vi "14.2 Bottle Check.vi"(8 "ErrI":errorcluster) -> (0 "ErrO":errorcluster)   [LabVIEW 2016]
uses:
  <vilib>/vision/Measure.llb/Straight Edge Options.ctl
  <vilib>/vision/Measure.llb/Straight Edge Process.ctl
  <vilib>/vision/Image Controls.llb/IMAQ Image.ctl
  <vilib>/vision/Measure.llb/Edge Options.ctl
  <vilib>/vision/Measure.llb/Edge Polarity.ctl
  <vilib>/vision/NI_Vision_Development_Module.lvlib
panel:
  out "Pass?":bool
  out "Liquied Level":dbl format="%.2f"
  in  "Line Fit Options":T1={"Number of Lines"=1, "Type"=enum."Best Edge Rake", "Min. Score"=10.0, "Max. Score"=1000.0, "Orientation"=0.0, "Angle Range"=45.0, "Angle Tolerance"=1.0, "Step Size"=7, "Min. SNR (db)"=0.0, "Min. Points (%)"=25.0, "Hough Iterations"=5} {"Min. Points (%)" min=0.0 max=100.0; "Min. SNR (db)" min=0.0; "Max. Score" min=0.0 max=1024.0; "Min. Score" min=0.0 max=1024.0 step=1.0}
  out "Image":T3(plugin-control)
  in  "Next":bool
  in  "Exit":bool
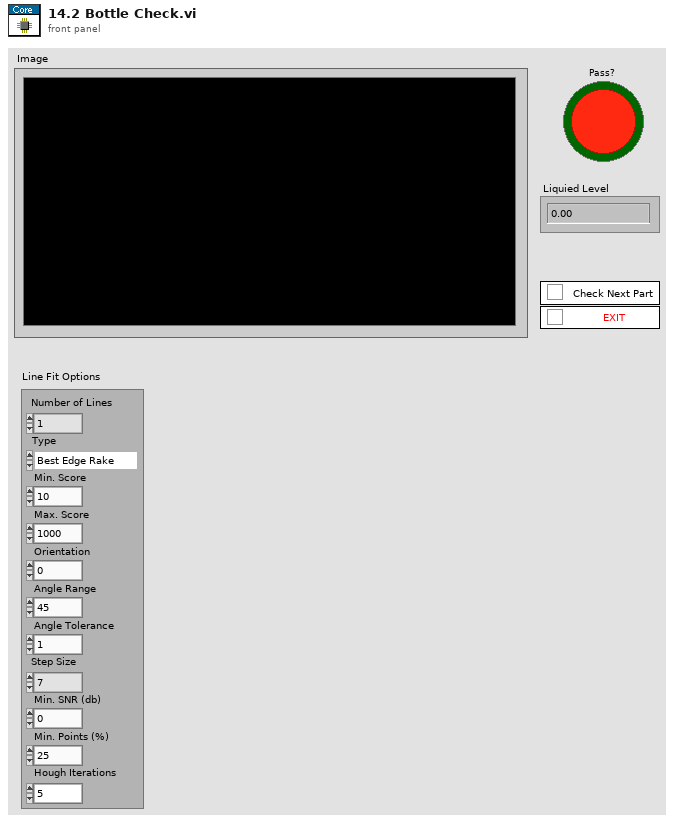
[diagram p1: front panel]
types:
  T1 = typedef "Straight Edge Options.ctl" = cluster{"Number of Lines":i32, "Type":T2, "Min. Score":dbl, "Max. Score":dbl, "Orientation":dbl, "Angle Range":dbl, "Angle Tolerance":dbl, "Step Size":u32, "Min. SNR (db)":dbl, "Min. Points (%)":dbl, "Hough Iterations":i32}
  T2 = typedef "Straight Edge Process.ctl" = enum32{"First Edge Rake", "Best Edge Rake", "Hough Edge Rake", "First Edge Projection", "Best Edge Projection"}
  T3 = typedef "IMAQ Image.ctl" = refnum<image>
  T4 = typedef "IMAQ Rectangle" = cluster{"Left":i32, "Top":i32, "Right":i32, "Bottom":i32, "Rotation":dbl}
  T5 = cluster{"Point1":cluster{"X":sgl, "Y":sgl}, "Point2":cluster{"X":sgl, "Y":sgl}}
  T6 = typedef "IMAQ Coordinate System" = cluster{"Reference System":cluster{"Origin":cluster{"X":sgl, "Y":sgl}, "Angle (deg)":sgl, "Axis Reference":u32}, "Measurement System":cluster{"Origin":cluster{"X":sgl, "Y":sgl}, "Angle (deg)":sgl, "Axis Reference":u32}}
  T7 = cluster{"Src":T3, "Dst":T3, "Parts":string[], "RefCoord":T6, "MsrCoord":T6, "MsrROI":T4, "RefLine":cluster{"Point1":cluster{"X":sgl, "Y":sgl}, "Point2":cluster{"X":sgl, "Y":sgl}}}
  T8 = typedef "Edge Options.ctl" = cluster{"Edge Polarity":T9, "Kernel Size":u32, "Width":u32, "Minimum Edge Strength":sgl, "Interpolation Type":enum32{"Zero Order", "Bilinear", "Quadratic", "Cubic", "Bilinear Fixed"}, "Data Processing Method":enum32{"Average", "Median"}}
  T9 = typedef "Edge Polarity.ctl" = u32
  T10 = cluster{"Direction":u16, "Primary Edge Options":T8, "Secondary Edge Options":T8, "Show Search Area":bool, "Show Search Lines":bool, "Show Edges Found":bool, "Show Result":bool, "Search Area Color":u32, "Search Lines Color":u32, "Edge Locations Color":u32, "Result Color":u32, "Overlay Group Name":string}
  T11 = typedef "ROI Descriptor" = cluster{"Global Rectangle":i32[], "Contours":cluster{"ID":enum32{"External", "Internal"}, "Type":u32, "Coordinates":i32[]}[]}
  T12 = cluster{"Search Direction":u32, "Edge Options":T8, "Show Search Area":bool, "Show Search Lines":bool, "Show Edges Found":bool, "Show Result":bool, "Search Area Color":u32, "Search Lines Color":u32, "Edge Locations Color":u32, "Result Color":u32, "Overlay Group Name":string}
  T13 = cluster{"Point1 (Pixels)":cluster{"X":sgl, "Y":sgl}, "Point2 (Pixels)":cluster{"X":sgl, "Y":sgl}, "Point1 (Real-World)":cluster{"X":sgl, "Y":sgl}, "Point2 (Real-World)":cluster{"X":sgl, "Y":sgl}, "Angle (Pixel)":dbl, "Angle (Real-World)":dbl, "Score":dbl, "Straightness":dbl, "Average SNR (db)":dbl, "Calibration Valid":bool}[]
  T14 = cluster{"Point1 (Pixels)":cluster{"X":sgl, "Y":sgl}, "Point2 (Pixels)":cluster{"X":sgl, "Y":sgl}, "Point1 (Real-World)":cluster{"X":sgl, "Y":sgl}, "Point2 (Real-World)":cluster{"X":sgl, "Y":sgl}, "Angle (Pixel)":dbl, "Angle (Real-World)":dbl, "Score":dbl, "Straightness":dbl, "Average SNR (db)":dbl, "Calibration Valid":bool}
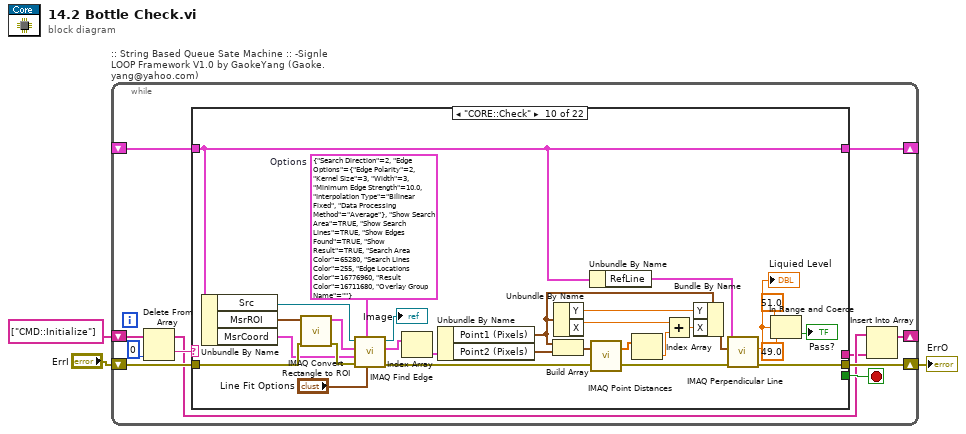
[diagram p0: block diagram]
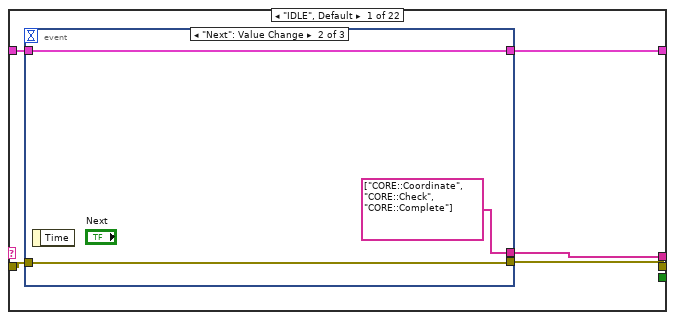
[diagram p2: hidden frame]
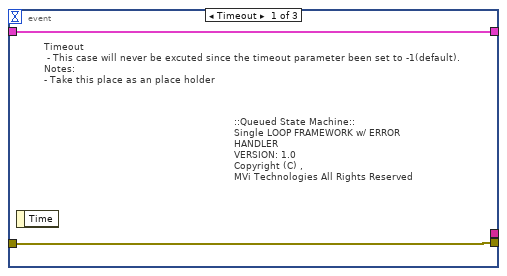
[diagram p3: hidden frame]
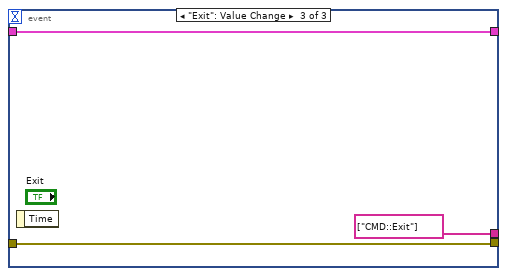
[diagram p4: hidden frame]
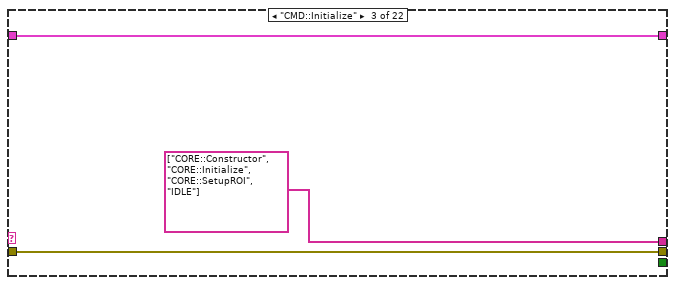
[diagram p6: hidden frame]
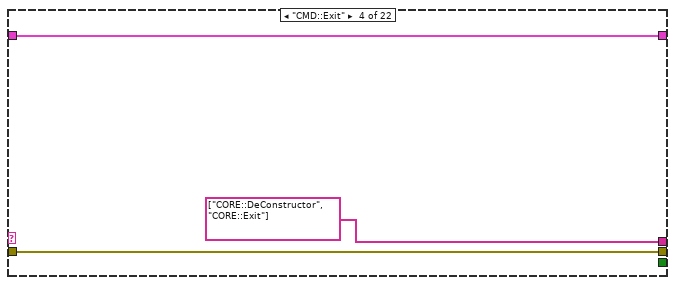
[diagram p7: hidden frame]
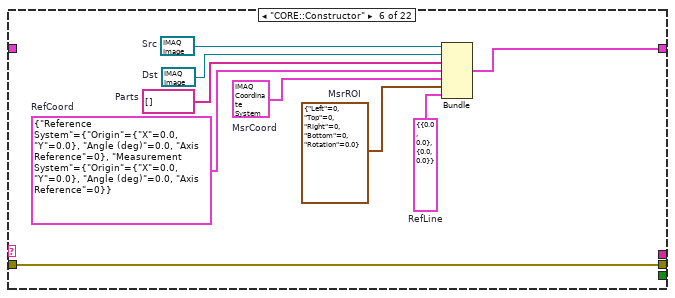
[diagram p9: hidden frame]
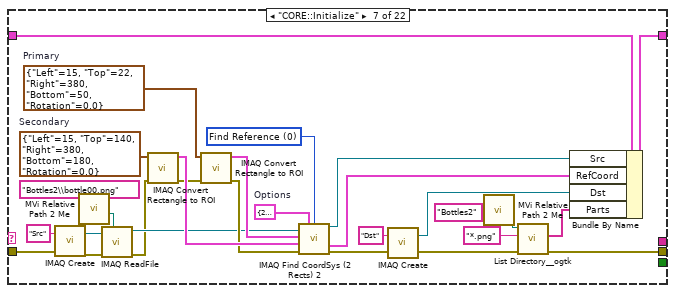
[diagram p10: hidden frame]
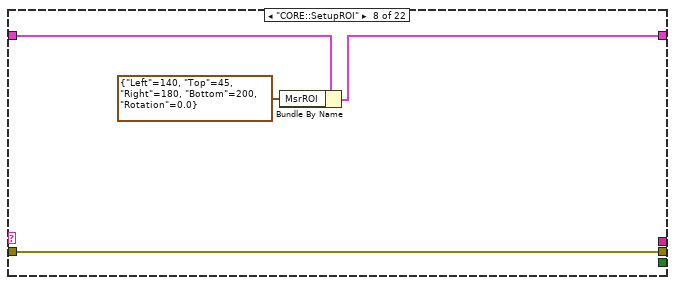
[diagram p11: hidden frame]
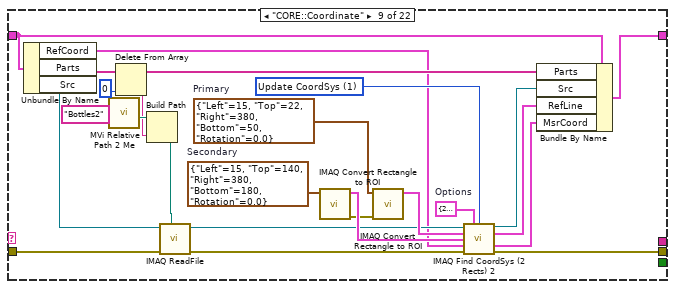
[diagram p12: hidden frame]
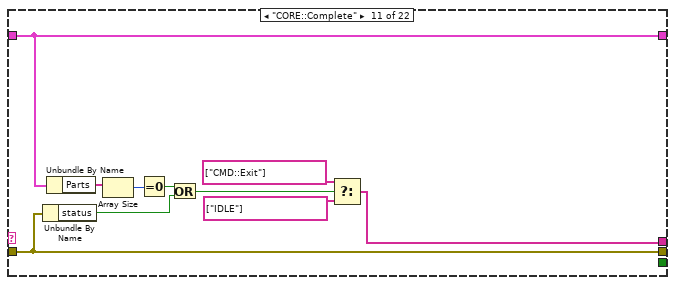
[diagram p13: hidden frame]
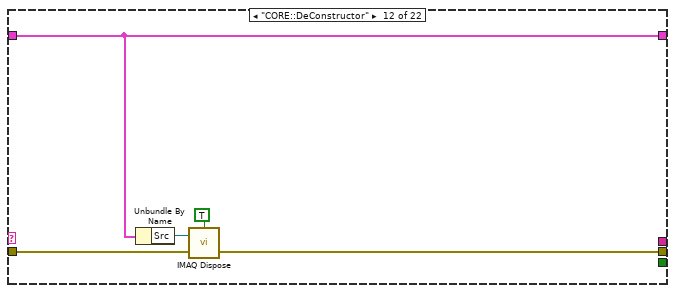
[diagram p14: hidden frame]
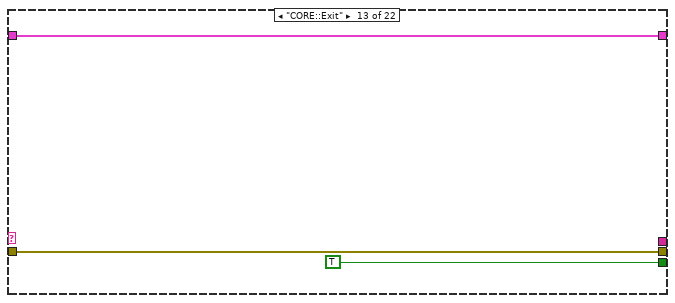
[diagram p15: hidden frame]
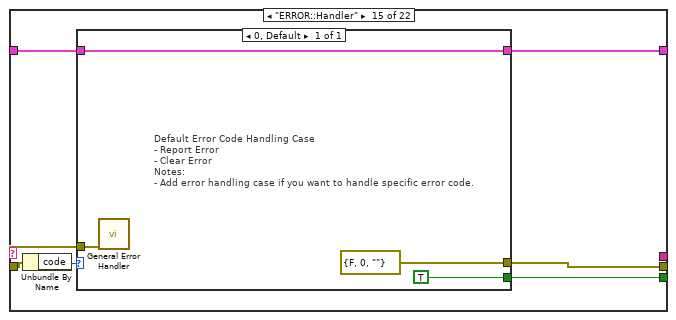
[diagram p17: hidden frame]
diagram:
  n1 = while ":: String Based Queue Sate Machine :: -Signle LOOP Framework V1.0 by GaokeYang (Gaoke.yang@yahoo.com)" {
    shift-right: [w11] -> w3
    shift-left: "ErrI" -> [w9]
    shift-right: [w13] -> _
    shift-left: _ -> [w12]
    shift-right: [w4] -> _
    shift-left: string[] ["CMD::Initialize"] -> [w10]
    stop <- w14 stop-if-true
    n2 = Delete From Array(array=w10, index=0) -> (deleted portion=w8:string, array with subset deleted=w6:string[])  [unwired: 1 in]
    n3 = case shown="\"CORE::Check\"" w8 {
      tunnel: [w18 w29 w31 w34 w37 w45 w64 w76 w84 w111 w139 w147 w149 w153 w156 w164 w166 w168 w171 w173 w175 w176] -> w11
      tunnel: [_ _ _ _ _ _ _ _ _ _ _ _ TRUE _ w155 _ _ _ _ _ _ _] -> w14
      tunnel: w9 -> [w19 w29 w31 w34 w37 w45 w68 w76 w99 w132 w139 w148 w149 w153 w154 w164 w166 w168 w171 w173 w175 w176]
      tunnel: [w16 w28 w32 w35 w36 w46 w72 w79 w96 w110 w140 w146 w150 w152 w157 w165 w167 w169 w170 w172 w174 w177] -> w13
      tunnel: w12 -> [w17 w28 w32 w35 w36 _ w73 w78 w97 w110 w140 w146 w150 w152 w158 w165 w167 w169 w170 w172 w174 w177]
      tunnel: [w15 _ string[] ["CORE::Constructor", "CORE::Initialize", "CORE::SetupROI", "IDLE"] string[] ["CORE::DeConstructor", "CORE::Exit"] _ _ _ _ _ _ w141 _ _ _ _ _ _ _ _ _ _ _] -> w5
      frame "IDLE", Default {
        n4 = event shown="[1] \"Next\": Value Change" {
          selector: _ -> [_ _ _]
          dyn-events: _ -> [_ _ _]
          timeout: _ -> [_ _ _]
          tunnel: [w21 w24 w27] -> w18
          tunnel: w19 -> [w21 w24 w27]
          tunnel: [w20 w23 w26] -> w16
          tunnel: w17 -> [w20 w23 w26]
          tunnel: [_ string[] ["CORE::Coordinate", "CORE::Check", "CORE::Complete"] string[] ["CMD::Exit"]] -> w15
          event Timeout {
            # "Timeout\n - This case will never be excuted since the timeout parameter been set to -1(default).\nNotes:\n- Take this place as an place holder"
            # "::Queued State Machine::\nSingle LOOP FRAMEWORK w/ ERROR HANDLER\nVERSION: 1.0\nCopyright (C) ,\nMVi Technologies All Rights Reserved"
            n5 = event-data() -> ()  [unwired: 1 in, 1 out]
          }
          event "Next": Value Change {
            n6 = event-data() -> ()  [unwired: 1 in, 1 out]
          }
          event "Exit": Value Change {
            n7 = event-data() -> ()  [unwired: 1 in, 1 out]
          }
        }
      }
      frame "-------- Commands ---------" {
      }
      frame "CMD::Initialize" {
      }
      frame "CMD::Exit" {
      }
      frame "------------ Core ------------" {
      }
      frame "CORE::Constructor" {
        w38 = T5 {"Point1"={"X"=0.0, "Y"=0.0}, "Point2"={"X"=0.0, "Y"=0.0}}  # RefLine
        w39 = T4 {"Left"=0, "Top"=0, "Right"=0, "Bottom"=0, "Rotation"=0.0}  # MsrROI
        w40 = T6 {"Reference System"={"Origin"={"X"=0.0, "Y"=0.0}, "Angle (deg)"=0.0, "Axis Reference"=0}, "Measurement System"={"Origin"={"X"=0.0, "Y"=0.0}, "Angle (deg)"=0.0, "Axis Reference"=0}}  # MsrCoord
        w41 = T6 {"Reference System"={"Origin"={"X"=0.0, "Y"=0.0}, "Angle (deg)"=0.0, "Axis Reference"=0}, "Measurement System"={"Origin"={"X"=0.0, "Y"=0.0}, "Angle (deg)"=0.0, "Axis Reference"=0}}  # RefCoord
        w44 = T3 refnum  # Dst
        w43 = string[] []  # Parts
        w42 = T3 refnum  # Src
        n8 = Bundle("Src"=w42, "Dst"=w44, "Parts"=w43, "RefCoord"=w41, "MsrCoord"=w40, "MsrROI"=w39, "RefLine"=w38) -> (w46:T7)  [unwired: 1 in]
      }
      frame "CORE::Initialize" {
        w56 = T4 {"Left"=15, "Top"=140, "Right"=380, "Bottom"=180, "Rotation"=0.0}  # Secondary
        w57 = T4 {"Left"=15, "Top"=22, "Right"=380, "Bottom"=50, "Rotation"=0.0}  # Primary
        w55 = T10 {"Direction"=2, "Primary Edge Options"={"Edge Polarity"=0, "Kernel Size"=3, "Width"=3, "Minimum Edge Strength"=10.0, "Interpolation Type"=enum."Bilinear Fixed", "Data Processing Method"=enum."Average"}, "Secondary Edge Options"={"Edge Polarity"=0, "Kernel Size"=3, "Width"=3, "Minimum Edge Strength"=10.0, "Interpolation Type"=enum."Bilinear Fixed", "Data Processing Method"=enum."Average"}, "Show Search Area"=TRUE, "Show Search Lines"=TRUE, "Show Edges Found"=TRUE, "Show Result"=TRUE, "Search Area Color"=65280, "Search Lines Color"=255, "Edge Locations Color"=14811391, "Result Color"=16711704, "Overlay Group Name"=""}  # Options
        w59 = u16 0 items=["Find Reference", "Update CoordSys"] ("Mode")
        n9 = call "IMAQ Create"("Image Name"="Src", "error in (no error)"=w68) -> ("Src"=w71:T3, "error out"=w69:errorcluster)  [unwired: 3 in]
        n10 = call "MVi Relative Path 2 Me.vi"("Relative Path"="Bottles2\\bottle00.png" ("name or relative path")) -> ("Appended Dir"=w70:path)  [unwired: 5 in, 1 out]
        n11 = call "IMAQ ReadFile"("File Path"=w70, "error in (no error)"=w69, "Image"=w71) -> ("error out"=w50:errorcluster, "Image Out"=w51:T3)  [unwired: 4 in, 3 out]
        n12 = call "IMAQ Convert Rectangle to ROI"("error in (no error)"=w50, "Rectangle"=w56) -> ("error out"=w54:errorcluster, "ROI Descriptor"=w58:T11)  [unwired: 7 in]
        n13 = call "IMAQ Convert Rectangle to ROI"("error in (no error)"=w54, "Rectangle"=w57) -> ("error out"=w53:errorcluster, "ROI Descriptor"=w52:T11)  [unwired: 7 in]
        n14 = call "IMAQ Find CoordSys (2 Rects) 2"("Image"=w51, "Options"=w55, "Mode"=w59, "Primary ROI Descriptor"=w52, "Secondary ROI Descriptor"=w58, "error in (no error)"=w53) -> ("Image Out"=w48:T3, "Coordinate System Out"=w47:T6, "error out"=w49:errorcluster)  [unwired: 5 in, 2 out]
        n15 = call "IMAQ Create"("Image Name"="Dst", "error in (no error)"=w49) -> ("Src"=w61:T3, "error out"=w62:errorcluster)  [unwired: 3 in]
        n16 = call "MVi Relative Path 2 Me.vi"("Relative Path"="Bottles2" ("name or relative path")) -> ("Appended Dir"=w66:path)  [unwired: 5 in, 1 out]
        n17 = call "List Directory__ogtk.vi"("error in (no error)"=w62, "pattern"="*.png", "directory path"=w66) -> ("error out"=w64:errorcluster, "file names"=w60:string[])  [unwired: 1 in, 2 out]
        n18 = Bundle By Name(cluster=w73, "Src"=w48, "RefCoord"=w47, "Dst"=w61, "Parts"=w60) -> (w72:T7)
      }
      frame "CORE::SetupROI" {
        n19 = Bundle By Name(cluster=w78, "MsrROI"=T4 {"Left"=140, "Top"=45, "Right"=180, "Bottom"=200, "Rotation"=0.0} ("Rectangle")) -> (w79:T7)
      }
      frame "CORE::Coordinate" {
        w90 = T4 {"Left"=15, "Top"=140, "Right"=380, "Bottom"=180, "Rotation"=0.0}  # Secondary
        w91 = T4 {"Left"=15, "Top"=22, "Right"=380, "Bottom"=50, "Rotation"=0.0}  # Primary
        w89 = T10 {"Direction"=2, "Primary Edge Options"={"Edge Polarity"=0, "Kernel Size"=3, "Width"=3, "Minimum Edge Strength"=10.0, "Interpolation Type"=enum."Bilinear Fixed", "Data Processing Method"=enum."Average"}, "Secondary Edge Options"={"Edge Polarity"=0, "Kernel Size"=3, "Width"=3, "Minimum Edge Strength"=10.0, "Interpolation Type"=enum."Bilinear Fixed", "Data Processing Method"=enum."Average"}, "Show Search Area"=TRUE, "Show Search Lines"=TRUE, "Show Edges Found"=TRUE, "Show Result"=TRUE, "Search Area Color"=65280, "Search Lines Color"=255, "Edge Locations Color"=14811391, "Result Color"=16711704, "Overlay Group Name"=""}  # Options
        w93 = u16 1 items=["Find Reference", "Update CoordSys"] ("Mode")
        n20 = Unbundle By Name(w97) -> ("RefCoord"=w82:T6, "Parts"=w95:string[], "Src"=w94:T3)
        n21 = call "MVi Relative Path 2 Me.vi"("Relative Path"="Bottles2" ("name or relative path")) -> ("Appended Dir"=w103:path)  [unwired: 5 in, 1 out]
        n22 = Delete From Array(array=w95, index=0) -> (deleted portion=w101:string, array with subset deleted=w98:string[])  [unwired: 1 in]
        n23 = Build Path(base path=w103, name or relative path=w101) -> (appended path=w100:path)
        n24 = call "IMAQ ReadFile"("File Path"=w100, "error in (no error)"=w99, "Image"=w94) -> ("error out"=w86:errorcluster, "Image Out"=w85:T3)  [unwired: 4 in, 3 out]
        n25 = call "IMAQ Convert Rectangle to ROI"("Rectangle"=w90) -> ("error out"=w88:errorcluster, "ROI Descriptor"=w92:T11)  [unwired: 8 in]
        n26 = call "IMAQ Convert Rectangle to ROI"("error in (no error)"=w88, "Rectangle"=w91) -> ("ROI Descriptor"=w87:T11)  [unwired: 7 in, 1 out]
        n27 = call "IMAQ Find CoordSys (2 Rects) 2"("Image"=w85, "Options"=w89, "Mode"=w93, "Primary ROI Descriptor"=w87, "Secondary ROI Descriptor"=w92, "Coordinate System In"=w82, "error in (no error)"=w86) -> ("Image Out"=w83:T3, "Main Axis"=w81:T5, "Coordinate System Out"=w80:T6, "error out"=w84:errorcluster)  [unwired: 4 in, 1 out]
        n28 = Bundle By Name(cluster=w97, "Parts"=w98, "Src"=w83, "RefLine"=w81, "MsrCoord"=w80) -> (w96:T7)
      }
      frame "CORE::Check" {
        w126 = T12 {"Search Direction"=2, "Edge Options"={"Edge Polarity"=2, "Kernel Size"=3, "Width"=3, "Minimum Edge Strength"=10.0, "Interpolation Type"=enum."Bilinear Fixed", "Data Processing Method"=enum."Average"}, "Show Search Area"=TRUE, "Show Search Lines"=TRUE, "Show Edges Found"=TRUE, "Show Result"=TRUE, "Search Area Color"=65280, "Search Lines Color"=255, "Edge Locations Color"=16776960, "Result Color"=16711680, "Overlay Group Name"=""}  # Options
        n29 = Unbundle By Name(w110) -> ("Src"=w133:T3, "MsrROI"=w130:T4, "MsrCoord"=w128:T6)
        n30 = call "IMAQ Convert Rectangle to ROI"("error in (no error)"=w132, "Rectangle"=w130) -> ("error out"=w131:errorcluster, "ROI Descriptor"=w129:T11)  [unwired: 7 in]
        n31 = call "IMAQ Find Edge"("Line Fit Options"="Line Fit Options", "Options"=w126, "error in (no error)"=w131, "Coordinate System"=w128, "ROI Descriptor"=w129, "Image"=w133) -> ("error out"=w121:errorcluster, "Straight Edges"=w124:T13, "Image Out"=→"Image":T3)  [unwired: 2 in, 1 out]
        n32 = Index Array(array=w124) -> (element=w123:T14)  [unwired: 1 in]
        n33 = Unbundle By Name(w123) -> ("Point1 (Pixels)"=w114:cluster{"X":sgl, "Y":sgl}, "Point2 (Pixels)"=w113:cluster{"X":sgl, "Y":sgl})
        n34 = Build Array(w114, w113) -> (w122:cluster{"X":sgl, "Y":sgl}[])
        n35 = Unbundle By Name(w114) -> ("Y"=w117:sgl, "X"=w120:sgl)
        n36 = Unbundle By Name(w110) -> ("RefLine"=w109:T5)
        n37 = call "IMAQ Point Distances"("Points"=w122, "error in (no error)"=w121) -> ("Distances"=w119:sgl[], "error out"=w112:errorcluster)  [unwired: 3 in]
        n38 = Index Array(array=w119) -> (element=w118:sgl)  [unwired: 1 in]
        n39 = Add(x=w120, y=w118) -> (x+y=w116:sgl)
        n40 = Bundle By Name(cluster=w114, "Y"=w117, "X"=w116) -> (w115:cluster{"X":sgl, "Y":sgl})
        n41 = call "IMAQ Perpendicular Line"("error in (no error)"=w112, "Point"=w115, "Line"=w109) -> ("error out"=w111:errorcluster, "Distance"=w108:dbl)  [unwired: 6 in, 1 out]
        "Liquied Level" <- w108
        n42 = In Range and Coerce(upper limit=51.0, x=w108, lower limit=49.0) -> (In Range?=→"Pass?":bool)  [unwired: 1 out]
      }
      frame "CORE::Complete" {
        n43 = Unbundle By Name(w139) -> ("status"=w135:bool)
        n44 = Unbundle By Name(w140) -> ("Parts"=w138:string[])
        n45 = Array Size(array=w138) -> (size(s)=w137:i32)
        n46 = Equal To 0?(x=w137) -> (x = 0?=w136:bool)
        n47 = Or(x=w136, y=w135) -> (x .or. y?=w134:bool)
        n48 = Select(t=string[] ["CMD::Exit"], s=w134, f=string[] ["IDLE"]) -> (s? t:f=w141:string[])
      }
      frame "CORE::DeConstructor" {
        n49 = Unbundle By Name(w146) -> ("Src"=w145:T3)
        n50 = call "IMAQ Dispose"("All Images? (No)"=TRUE, "Image"=w145, "error in (no error)"=w148) -> ("error out"=w147:errorcluster)  [unwired: 3 in]
      }
      frame "CORE::Exit" {
      }
      frame "-------- Error Handle--------" {
      }
      frame "ERROR::Handler" {
        n51 = Unbundle By Name(w154) -> ("code"=w159:i32)
        n52 = case shown="0, Default" w159 {
          tunnel: [w163] -> w157
          tunnel: w158 -> [w163]
          tunnel: [errorcluster {"status"=FALSE, "code"=0, "source"=""} ("error out")] -> w156
          tunnel: [TRUE] -> w155
          tunnel: w154 -> [w161]
          frame 0, Default {
            # "Default Error Code Handling Case\n- Report Error\n- Clear Error \nNotes:\n- Add error handling case if you want to handle specific error code."
            n53 = call <vilib>:"General Error Handler.vi"("error in (no error)"=w161) -> ()  [unwired: 10 in, 5 out]
          }
        }
      }
      frame "------------  GUI  ------------" {
      }
      frame "GUI::Initialize" {
      }
      frame "GUI::SetCusor" {
      }
      frame "GUI::SetMenu" {
      }
      frame "------------ USER -----------" {
      }
      frame "USER::Case1" {
      }
      frame "USER::Case2" {
      }
    }
    n54 = Insert Into Array(array=w6, new element=w5) -> (w4:string[])  [unwired: 1 in]
  }
  "ErrO" <- w3
